vi "App_Main Insert Subpanel.vi"(8 "error in":errorcluster, 11 "VI Name":string) -> (0 "error out":errorcluster)   [LabVIEW 2018, in "Application 1.lvlib"]
uses:
  Application 1.lvlib
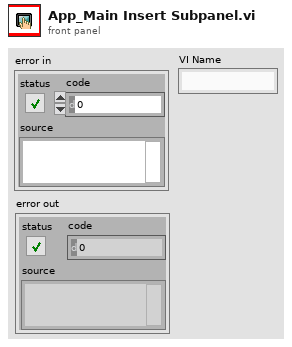
[diagram p1: front panel]
types:
  T1 = typedef "Application 1.lvlib/App_Main Data.ctl" = cluster{"VI Refnum":refnum<vi>, "Subpanel":refnum<vi>, "Connection ID":refnum<k5>, "Meta data":T2[], "Main Queue":T4, "User Data":T5}
  T2 = typedef "stm_MetaElement.ctl" = cluster{"Name":T3}
  T3 = typedef "stm_MetaDataElement.ctl" = string
  T4 = typedef "Application 1.lvlib/App_Main Queue.ctl" = cluster{"Main Loop Queue":refnum<queue>}
  T5 = typedef "User Data.ctl" = cluster{"Name":string, "Email":string, "Phone Number":string, "User Picture":u32[][], "Last Login Time":timestamp}
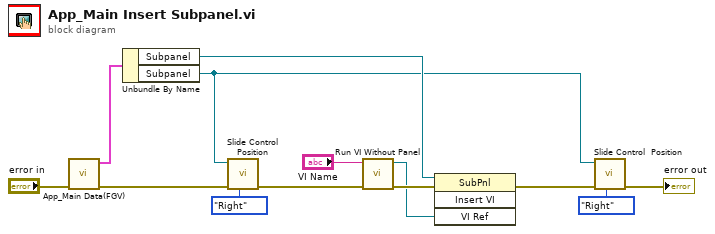
[diagram p0: block diagram]
diagram:
  n1 = call "App_Main Data(FGV).vi"("error in"="error in") -> ("error out"=w12:errorcluster, "Main Data Out"=w11:T1)  [unwired: 9 in]
  n2 = Unbundle By Name(w11) -> ("Subpanel"=w7:refnum<vi>, "Subpanel"=w2:refnum<vi>)
  n3 = call "Slide Control  Position.vi"("Direction"=enum16{"Right", "Left", "Down", "Up"}."Right", "error in"=w12, "Ctl Refnum"=w2) -> ("error out"=w9:errorcluster)  [unwired: 8 in]
  n4 = call "Run VI Without Panel.vi"("error in"=w9, "VI Name"="VI Name") -> ("error out"=w6:errorcluster, "vi reference"=w5:refnum<vi>)  [unwired: 8 in]
  n5 = invoke class="SubPnl" method="Insert VI"(reference=w7, error in=w6, "VI Ref"=w5) -> (error out=w3:errorcluster)  [unwired: 1 in, 3 out]
  n6 = call "Slide Control  Position.vi"("Direction"=enum16{"Right", "Left", "Down", "Up"}."Right", "error in"=w3, "Ctl Refnum"=w2) -> ("error out"=→"error out":errorcluster)  [unwired: 8 in]
